vi "tcp vi port.vi"() -> (3 "port":u16)   [LabVIEW 2013]
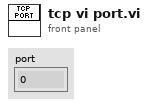
[diagram p1: front panel]
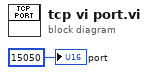
[diagram p0: block diagram]
diagram:
  "port" <- u16 15050 ("port")
